vi "cluster 2.vi"() -> ()   [LabVIEW 2018]
panel:
  out "Total using sigma":dbl
  out "Cluster 2":T1
  in  "Cluster":T1
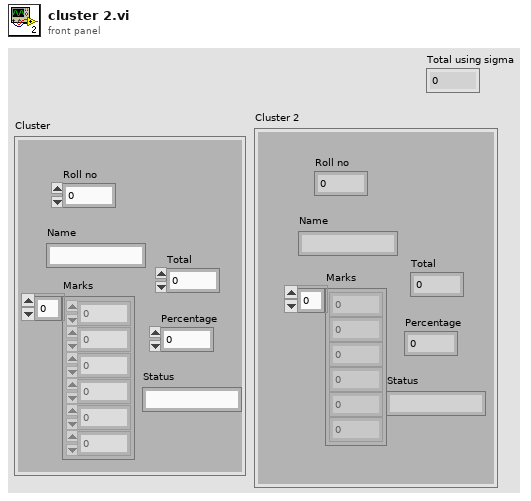
[diagram p1: front panel]
types:
  T1 = cluster{"Roll no":dbl, "Name":string, "Marks":dbl[], "Total":dbl, "Percentage":dbl, "Status":string}
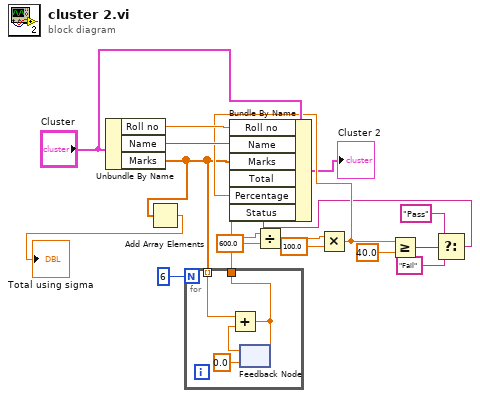
[diagram p0: block diagram]
diagram:
  n1 = Unbundle By Name("Cluster") -> ("Roll no"=w16:dbl, "Name"=w15:string, "Marks"=w2:dbl[])
  n2 = Add Array Elements(numeric array=w2) -> (sum=→"Total using sigma":dbl)
  n3 = for {
    N: 6 -> [_]
    tunnel: w2 -> [w21] mode=indexing
    tunnel: [w18] -> w13
    n4 = feedback #1(0.0) -> (w20:dbl)
    n5 = Add(x=w21, y=w20) -> (x+y=w18:dbl)
    n6 = feedback-in #1(w18) -> ()
  }
  n7 = Divide(x=w13, y=600.0) -> (x/y=w11:dbl)
  n8 = Multiply(x=w11, y=100.0) -> (x*y=w8:dbl)
  n9 = Greater Or Equal?(x=w8, y=40.0) -> (x >= y?=w9:bool)
  n10 = Select(t="Pass", s=w9, f="Fail") -> (s? t:f=w4:string)
  n11 = Bundle By Name(cluster="Cluster", "Roll no"=w16, "Name"=w15, "Marks"=w2, "Total"=w13, "Percentage"=w8, "Status"=w4) -> (→"Cluster 2":T1)
